vi "freq_magnitude_to_XY.vi"(8 "error in (no error)":errorcluster, 11 "magnitude []":cluster{"f0":dbl, "df":dbl, "magnitude":dbl[]}[](array[cluster])) -> (0 "error out":errorcluster, 3 "freq_magnitude_XY":cluster{dbl[], "magnitude":dbl[]}[](array[cluster]))   [LabVIEW 2016]
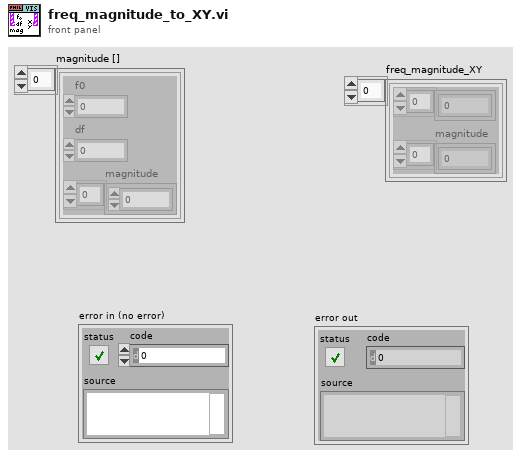
[diagram p1: front panel]
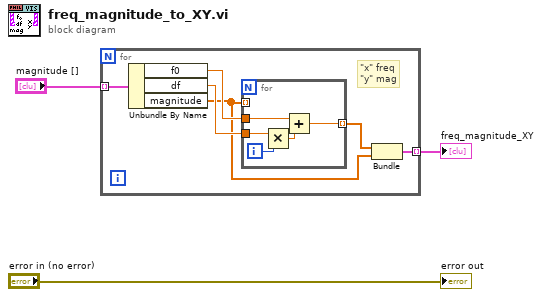
[diagram p0: block diagram]
diagram:
  n1 = for {
    tunnel: "magnitude []" -> [w9] mode=indexing
    tunnel: [w4] -> w2 mode=indexing
    # "\"x\" freq\n\"y\" mag"
    n2 = Unbundle By Name(w9) -> ("f0"=w7:dbl, "df"=w8:dbl, "magnitude"=w5:dbl[])
    n3 = for {
      tunnel: w5 -> [_] mode=indexing
      tunnel: w8 -> [w14]
      tunnel: w7 -> [w12]
      tunnel: [w10] -> w6 mode=indexing
      i -> [w13]
      n4 = Multiply(x=w14, y=w13) -> (x*y=w11:dbl)
      n5 = Add(x=w12, y=w11) -> (x+y=w10:dbl)
    }
    n6 = Bundle(w6, "magnitude"=w5) -> (w4:cluster{dbl[], "magnitude":dbl[]})  [unwired: 1 in]
  }
  "freq_magnitude_XY" <- w2
  "error out" <- "error in (no error)"
